vi "Update Connection.vi"(7 "new channel":string, 8 "error in (no error)":errorcluster, 9 "connected channel":string, 10 "common channel":string, 11 "switch":refnum<k15>) -> (0 "error out":errorcluster)   [LabVIEW 2023, in "FPT_SParam_Switching.lvclass"]
uses:
  FPT_SParam_Switching.lvclass
  FPT_SParam_Switching.lvclass/FPT_SParam_Switching.ctl
  <instrlib>/niSwitch/niSwitch.llb/niSwitch Connect Channels (Single).vi
  <instrlib>/niSwitch/niSwitch.llb/niSwitch Disconnect Channels (Single).vi
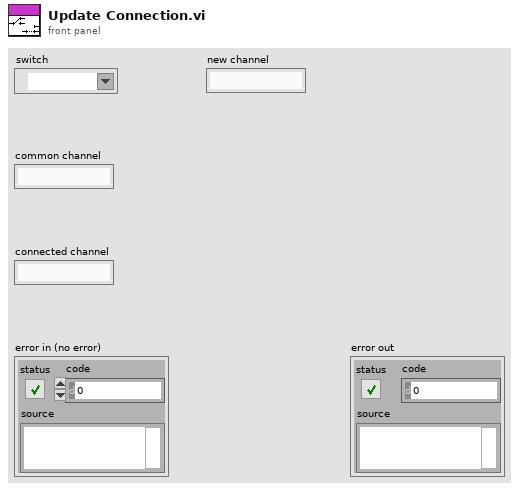
[diagram p1: front panel]
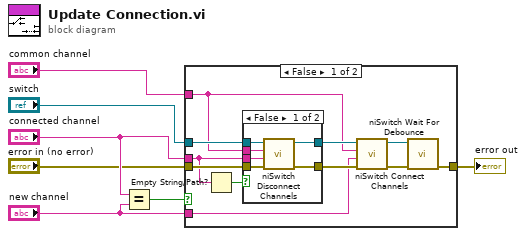
[diagram p0: block diagram]
diagram:
  n1 = Equal?(x="connected channel", y="new channel") -> (x = y?=w1:bool)
  n2 = case shown="False" w1 {
    tunnel: "error in (no error)" -> [w16 w27]
    tunnel: "switch" -> [w15 _]
    tunnel: "connected channel" -> [w8 _]
    tunnel: "common channel" -> [w10 _]
    tunnel: "new channel" -> [w11 _]
    tunnel: [w12 w27] -> w7
    frame False {
      n3 = Empty String/Path?(string/path=w8) -> (empty?=w9:bool)
      n4 = case shown="False" w9 {
        tunnel: w16 -> [w24 w26]
        tunnel: w15 -> [w23 w25]
        tunnel: [w22 w26] -> w14
        tunnel: [w21 w25] -> w13
        tunnel: w10 -> [w20 _]
        tunnel: w8 -> [w19 _]
        frame False {
          n5 = call-poly <instrlib>:"niSwitch Disconnect Channels.vi"("error in (no error)"=w24, "channel 2"=w19, "channel 1"=w20, "instrument handle"=w23) -> ("error out"=w22:errorcluster, "instrument handle out"=w21:refnum<k15>)  [unwired: 6 in]
        }
        frame True {
        }
      }
      n6 = call-poly <instrlib>:"niSwitch Connect Channels.vi"("error in (no error)"=w14, "channel 2"=w11, "channel 1"=w10, "instrument handle"=w13) -> ("error out"=w18:errorcluster, "instrument handle out"=w17:refnum<k15>)  [unwired: 6 in]
      n7 = call <instrlib>:"niSwitch Wait For Debounce.vi"("error in (no error)"=w18, "instrument handle"=w17) -> ("error out"=w12:errorcluster)  [unwired: 1 in, 8 out]
    }
    frame True {
    }
  }
  "error out" <- w7
